vi "find_stage_orientation.vi"(9 "Home pose":dbl[](array[numeric])=[0.25469575119784055, -16.45995133588347, 3.732397870471535, 0.0, 0.0, 0.0] format="%#.3f", 10 "Point selector":T3={"Pose mode"=enum."Light", "Light number"=5} {"Light number" min=0 max=5}, 11 "Override":T1) -> (1 "Axis scale errors (percent)":sgl[](array[numeric]) format="%#_4p", 2 "Stage pose (rotation only)":T2 format="%#_3f", 3 "Axis errors (radians)":dbl[](array[numeric]) format="%#_4p")   [LabVIEW 2013]
uses:
  calibration/point_selector.ctl
  <vilib>/Analysis/Matrix/Datatypes/RealMatrix.ctl
  ui_override_opts.ctl
  utilities/labview/norm_vec_single.vi
  <vilib>/Analysis/baseanly.llb/Real Dot Product.vi
  <vilib>/Analysis/Matrix/Numeric/Conversions/Array To Matrix - RA2.vi
  utilities/labview/norm_vec.vi
  <vilib>/Analysis/Matrix/Numeric/Conversions/Array To Matrix - RA.vi
  <vilib>/Analysis/Matrix/NI_Matrix.lvlib
  <vilib>/Analysis/NI_AALBase.lvlib
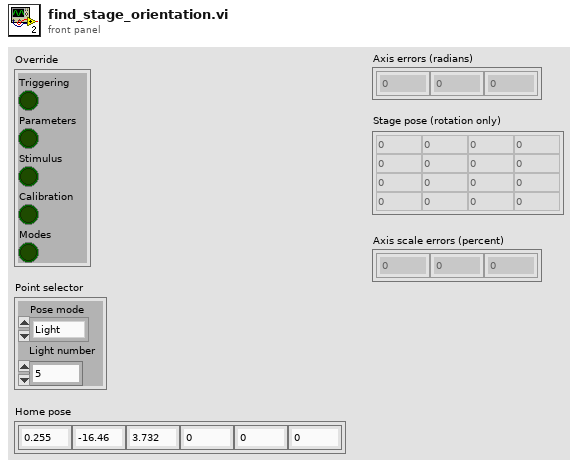
[diagram p1: front panel]
types:
  T1 = typedef "ui_override_opts.ctl" = cluster{"Triggering":bool, "Parameters":bool, "Stimulus":bool, "Calibration":bool, "Modes":bool}
  T2 = typedef "NI_Matrix.lvlib/RealMatrix.ctl" = dbl[][]
  T3 = typedef "point_selector.ctl" = cluster{"Pose mode":enum16{"Light", "Handle", "Output"}, "Light number":i32}
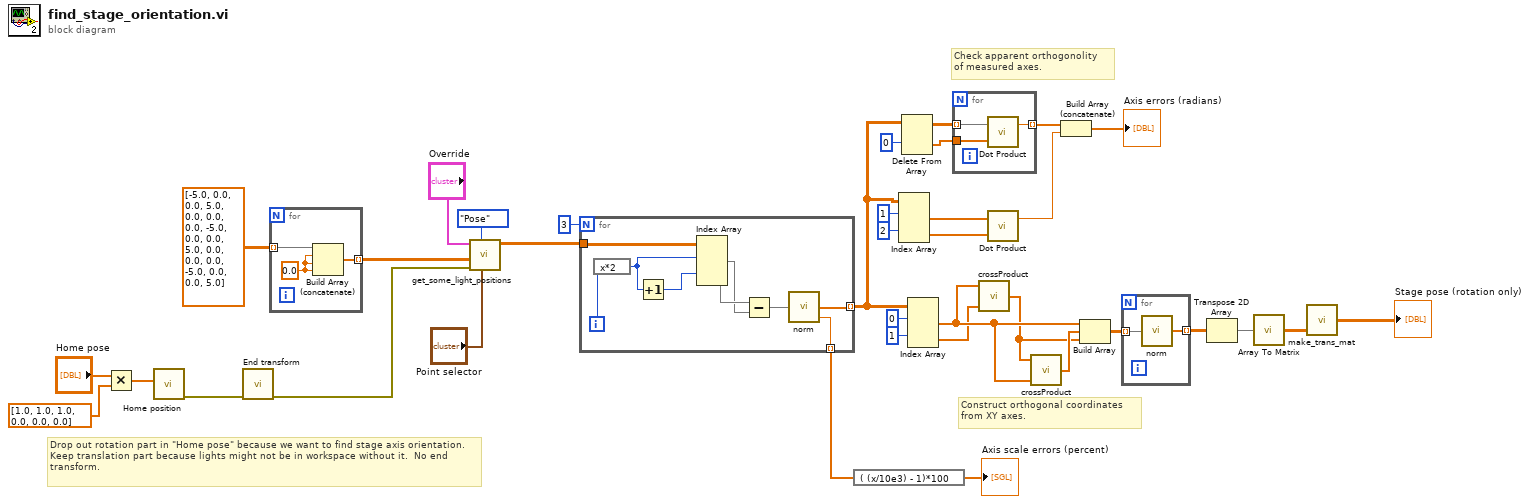
[diagram p0: block diagram]
diagram:
  # "Drop out rotation part in \"Home pose\" because we want to find stage axis orientation.  Keep translation part because lights might not be in workspace without it.  No end transform."
  # "Check apparent orthogonolity\nof measured axes."
  # "Construct orthogonal coordinates\nfrom XY axes."
  n1 = Multiply(x="Home pose", y=dbl[] [1.0, 1.0, 1.0, 0.0, 0.0, 0.0]) -> (x*y=w6:dbl[])
  n2 = call "Home position.vi"("Home position"=w6) -> ("error out"=w5:errorcluster)  [unwired: 10 in]
  n3 = call "End transform.vi"("error in"=w5) -> ("error out"=w4:errorcluster)  [unwired: 10 in]
  n4 = for {
    tunnel: dbl[][] [[-5.0, 0.0, 0.0], [5.0, 0.0, 0.0], [0.0, -5.0, 0.0], [0.0, 5.0, 0.0], [0.0, 0.0, -5.0], [0.0, 0.0, 5.0]] ("Sequence") -> [w38] mode=indexing
    tunnel: [w37] -> w10 mode=indexing
    w39 = 0.0
    n5 = Build Array (concatenate)(w38, w39, w39, w39) -> (w37:dbl[])
  }
  n6 = call "get_some_light_positions.vi"("Point selector"="Point selector", "Position mode"=enum16{"Absolute axis", "Relative axis", "Pose"}."Pose", "error in"=w4, "Sequence"=w10, "Override"="Override") -> ("Light positions"=w36:sgl[][])  [unwired: 4 in, 2 out]
  n7 = for {
    N: 3 -> [_]
    tunnel: w36 -> [w48]
    tunnel: [w42] -> w30 mode=indexing
    tunnel: [w40] -> w3 mode=indexing
    i -> [w45]
    n8 = expression code="x*2"(w45) -> (w47:i32)
    n9 = Increment(x=w47) -> (x+1=w46:i32)
    n10 = Index Array(array=w48, index (row) #1=w47, index (row) #2=w46) -> (element #1=w43:sgl[], element #2=w44:sgl[])  [unwired: 2 in]
    n11 = Subtract(x=w44, y=w43) -> (x-y=w41:sgl[])
    n12 = call-poly "norm.vi"("vector"=w41) -> ("magnitude"=w40:sgl, "normalized vector"=w42:sgl[])  [unwired: 3 in]
  }
  n13 = expression code="( (x/10e3) - 1)*100"(w3) -> (→"Axis scale errors (percent)":sgl[])
  n14 = Index Array(array=w30, index (row) #1=1 ("index (row)"), index (row) #2=2 ("index (row)")) -> (element #1=w31:sgl[], element #2=w32:sgl[])  [unwired: 2 in]
  n15 = Delete From Array(array=w30, index (row)=0) -> (deleted portion=w27:sgl[], array with subset deleted=w26:sgl[][])  [unwired: 2 in]
  n16 = Index Array(array=w30, index (row) #1=0 ("index (row)"), index (row) #2=1 ("index (row)")) -> (element #1=w23:sgl[], element #2=w16:sgl[])  [unwired: 2 in]
  n17 = for {
    tunnel: w26 -> [w51] mode=indexing
    tunnel: w27 -> [w50]
    tunnel: [w49] -> w34 mode=indexing
    n18 = call-poly <vilib>:"Dot Product.vi"("Y Vector"=w50, "X Vector"=w51) -> ("X * Y"=w49:dbl)  [unwired: 1 out]
  }
  n19 = call "crossProduct.vi"("B"=w16, "A"=w23) -> ("A x B"=w15:dbl[])  [unwired: 3 in]
  n20 = call-poly <vilib>:"Dot Product.vi"("Y Vector"=w32, "X Vector"=w31) -> ("X * Y"=w33:dbl)  [unwired: 1 out]
  n21 = call "crossProduct.vi"("B"=w23, "A"=w15) -> ("A x B"=w17:dbl[])  [unwired: 3 in]
  n22 = Build Array (concatenate)(w34, w33) -> (→"Axis errors (radians)":dbl[])
  n23 = Build Array(w23, w17, w15) -> (w21:dbl[][])
  n24 = for {
    tunnel: w21 -> [w52] mode=indexing
    tunnel: [w53] -> w22 mode=indexing
    n25 = call-poly "norm.vi"("vector"=w52) -> ("normalized vector"=w53:dbl[])  [unwired: 3 in, 1 out]
  }
  n26 = Transpose 2D Array(2D array=w22) -> (transposed array=w20:dbl[][])
  n27 = call-poly <vilib>:"Array To Matrix.vi"("Real 2D Array"=w20) -> ("Real Matrix"=w18:T2)
  n28 = call "make_trans_mat.vi"("Rotation"=w18) -> ("Transform"=→"Stage pose (rotation only)":T2)  [unwired: 4 in]
